vi "Current State Status.vi"(8 "error in (no error)":errorcluster, 10 "State Status":T1, 11 "Command Actor in":refnum<class "Command Actor.lvclass">) -> (0 "error out":errorcluster, 3 "Command Actor out":refnum<class "Command Actor.lvclass">)   [LabVIEW 2013, in "Command Actor.lvlib" / "Command Actor.lvclass"]
uses:
  Command Actor.lvclass
  Command/State Status.ctl
  Command States/Command States.lvclass
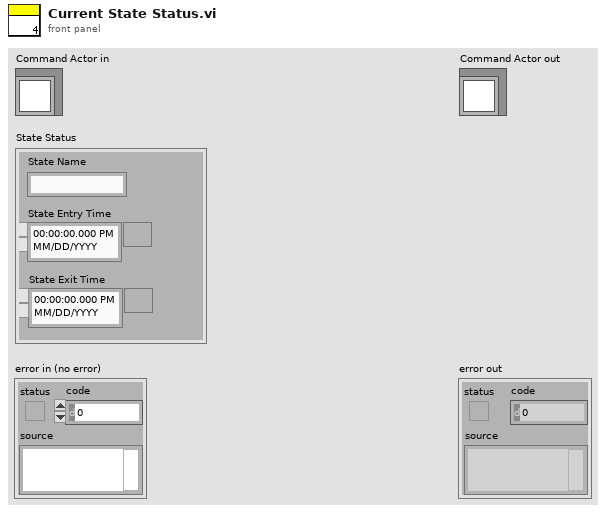
[diagram p1: front panel]
types:
  T1 = typedef "Command Actor.lvlib/Command States.lvclass/State Status.ctl" = cluster{"State Name":string, "State Entry Time":timestamp, "State Exit Time":timestamp}
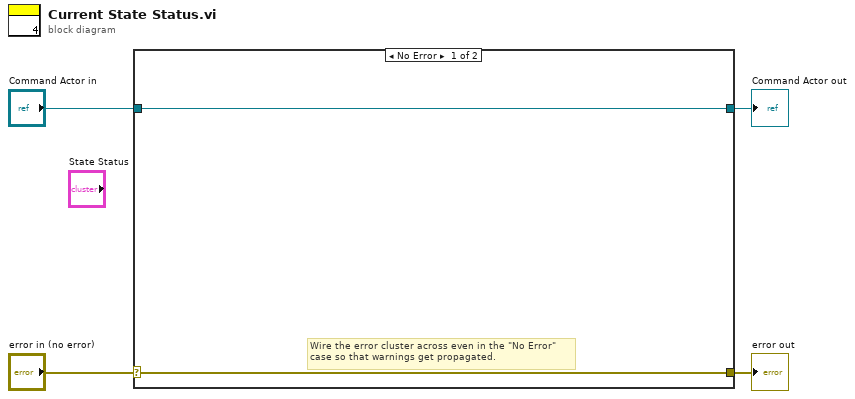
[diagram p0: block diagram]
diagram:
  n1 = case shown="No Error" "error in (no error)" {
    selector: "error in (no error)" -> [w5 w8]
    tunnel: [w5 w8] -> w3
    tunnel: [w6 w7] -> w1
    tunnel: "Command Actor in" -> [w6 w7]
    frame No Error {
      # "Wire the error cluster across even in the \"No Error\"\ncase so that warnings get propagated."
    }
    frame Error {
    }
  }
  "error out" <- w3
  "Command Actor out" <- w1
